vi "pololucontrol.vi"(6 "open":bool) -> ()   [LabVIEW 2012]
uses:
  <vilib>/DAQmx/write.llb/DAQmx Write (Digital Wfm 1Chan NSamp).vi
  <vilib>/DAQmx/create/channels.llb/DAQmx Create Channel (DO-Digital Output).vi
  <vilib>/DAQmx/configure/timing.llb/DAQmx Timing (Sample Clock).vi
  <vilib>/Waveform/DWDTOps.llb/DWDT Analog to Digital.vi
  <vilib>/Waveform/DWDTOps.llb/DWDT Uncompress Digital.vi
  <vilib>/DAQmx/miscellaneous.llb/DAQmx Fill In Error Info.vi
  <vilib>/measure/NI_MABase.lvlib
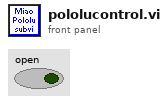
[diagram p1: front panel]
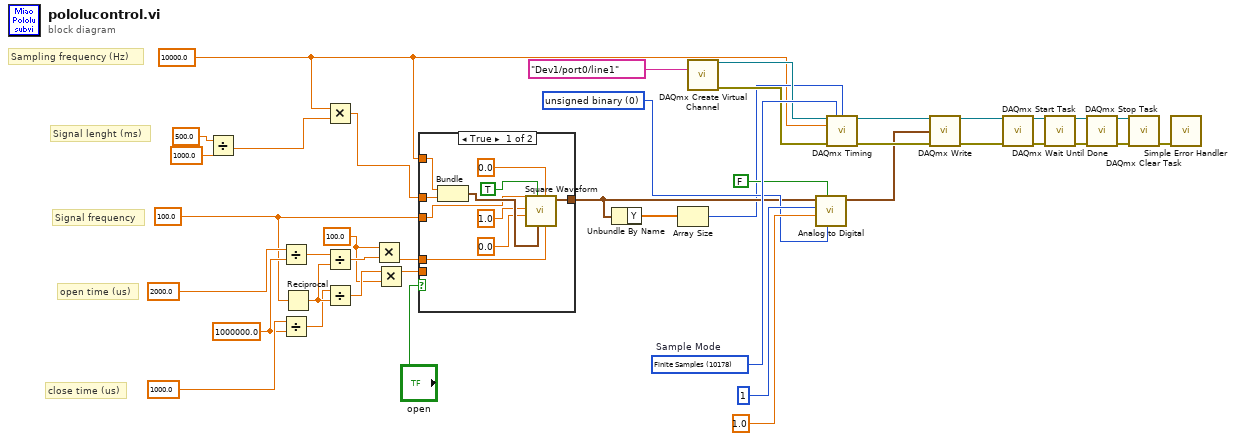
[diagram p0: block diagram]
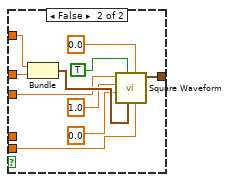
[diagram p2: hidden frame]
diagram:
  w18 = 100.0 ("frequency of command (Hz)")
  w1 = 100.0 ("y")
  w19 = 1000000.0 ("y")
  w6 = 10000.0 ("element")
  w28 = u16 0 items=["unsigned binary", "offset binary", "2's complement"] ("data format (offset binary)")
  w35 = 10178 items=["Finite Samples"=10178, "Continuous Samples"=10123, "Hardware Timed Single Point"=12522]  # Sample Mode
  # "close time (us)"
  # "open time (us)"
  # "Signal frequency"
  # "Signal lenght (ms)"
  # "Sampling frequency (Hz)"
  n1 = Divide(x=500.0 ("length of command (ms)"), y=1000.0) -> (x/y=w7:dbl)
  n2 = Divide(x=2000.0 ("open time (us)"), y=w19) -> (x/y=w17:dbl)
  n3 = Divide(x=1000.0 ("close time (us)"), y=w19) -> (x/y=w14:dbl)
  n4 = Reciprocal(x=w18) -> (1/x=w15:dbl)
  n5 = Multiply(x=w6, y=w7) -> (x*y=w5:dbl)
  n6 = Divide(x=w17, y=w15) -> (x/y=w16:dbl)
  n7 = Divide(x=w14, y=w15) -> (x/y=w13:dbl)
  n8 = Multiply(x=w1, y=w16) -> (x*y=w2:dbl)
  n9 = Multiply(x=w13, y=w1) -> (x*y=w3:dbl)
  n10 = case shown="True" "open" {
    tunnel: w5 -> [w50 w52]
    tunnel: w18 -> [w47 w58]
    tunnel: w2 -> [w46 _]
    tunnel: w6 -> [w43 w55]
    tunnel: [w42 w54] -> w11
    tunnel: w3 -> [_ w53]
    frame True {
      n11 = Bundle("element"=w43, w50) -> (w51:cluster{"element":dbl, dbl})  [unwired: 1 in]
      n12 = call <vilib>:"Square Waveform.vi"("duty cycle (%)"=w46, "offset"=0.0, "sampling info"=w51, "reset signal"=TRUE, "phase"=0.0, "amplitude"=1.0, "frequency"=w47) -> ("signal out"=w42:waveform(dbl))  [unwired: 3 in, 1 out]
    }
    frame False {
      n13 = Bundle("element"=w55, w52) -> (w61:cluster{"element":dbl, dbl})  [unwired: 1 in]
      n14 = call <vilib>:"Square Waveform.vi"("duty cycle (%)"=w53, "offset"=0.0, "sampling info"=w61, "reset signal"=TRUE, "phase"=0.0, "amplitude"=1.0, "frequency"=w58) -> ("signal out"=w54:waveform(dbl))  [unwired: 3 in, 1 out]
    }
  }
  n15 = Unbundle By Name(w11) -> ("Y"=w10:dbl[])
  n16 = Array Size(array=w10) -> (size(s)=w9:i32)
  n17 = call-poly <vilib>:"DAQmx Create Virtual Channel.vi"("lines"=tag "Dev1/port0/line1" ("Line(s)")) -> ("task out"=w33:refnum<k21>, "error out"=w34:errorcluster)  [unwired: 13 in]
  n18 = call-poly <vilib>:"Analog to Digital.vi"("data format (offset binary)"=w28, "compress digital (T)"=FALSE, "full-scale range (pk-pk)"=1.0, "resolution (16 bit)"=1, "analog waveform"=w11) -> ("digital waveform"=w4:digitalwaveform)  [unwired: 3 in, 3 out]
  n19 = call-poly <vilib>:"DAQmx Timing.vi"("task/channels in"=w33, "sample mode"=w35, "samples per channel"=w9, "rate"=w6, "error in"=w34) -> ("task out"=w40:refnum<k21>, "error out"=w41:errorcluster)  [unwired: 9 in]
  n20 = call-poly <vilib>:"DAQmx Write.vi"("task/channels in"=w40, "data"=w4, "error in"=w41) -> ("task out"=w38:refnum<k21>, "error out"=w39:errorcluster)  [unwired: 10 in, 1 out]
  n21 = call <vilib>:"DAQmx Start Task.vi"("task/channels in"=w38, "error in"=w39) -> ("task out"=w26:refnum<k21>, "error out"=w24:errorcluster)  [unwired: 12 in]
  n22 = call <vilib>:"DAQmx Wait Until Done.vi"("task/channels in"=w26, "error in"=w24) -> ("task out"=w25:refnum<k21>, "error out"=w23:errorcluster)  [unwired: 12 in]
  n23 = call <vilib>:"DAQmx Stop Task.vi"("task/channels in"=w25, "error in"=w23) -> ("task out"=w37:refnum<k21>, "error out"=w36:errorcluster)  [unwired: 12 in]
  n24 = call <vilib>:"DAQmx Clear Task.vi"("task in"=w37, "error in"=w36) -> ("error out"=w31:errorcluster)  [unwired: 13 in]
  n25 = call <vilib>:"Simple Error Handler.vi"("error in (no error)"=w31) -> ()  [unwired: 4 in, 5 out]
